vi "FEA_Model_Element_Matrix.vi"(11 "FEA_Model in":refnum<class "FEA_Model.lvclass">) -> (3 "FEA_Model out":refnum<class "FEA_Model.lvclass">)   [LabVIEW 2021, in "FEA_Model.lvclass"]
uses:
  FEA_Model.lvclass
  FEA_Model.lvclass/FEA_Model.ctl
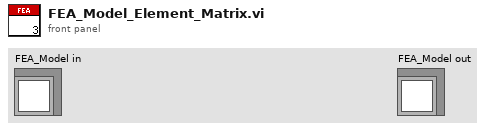
[diagram p1: front panel]
types:
  T1 = cluster{"beam_length":dbl, "youngs_modulus":dbl, "torsion_spring":dbl, "beam_height":dbl, "beam_width":dbl, "beam_density":dbl, "number_of_FEA_nodes":i32, "accelerometer_mass":dbl, "M Matrix":dbl[][], "K Matrix":dbl[][]}
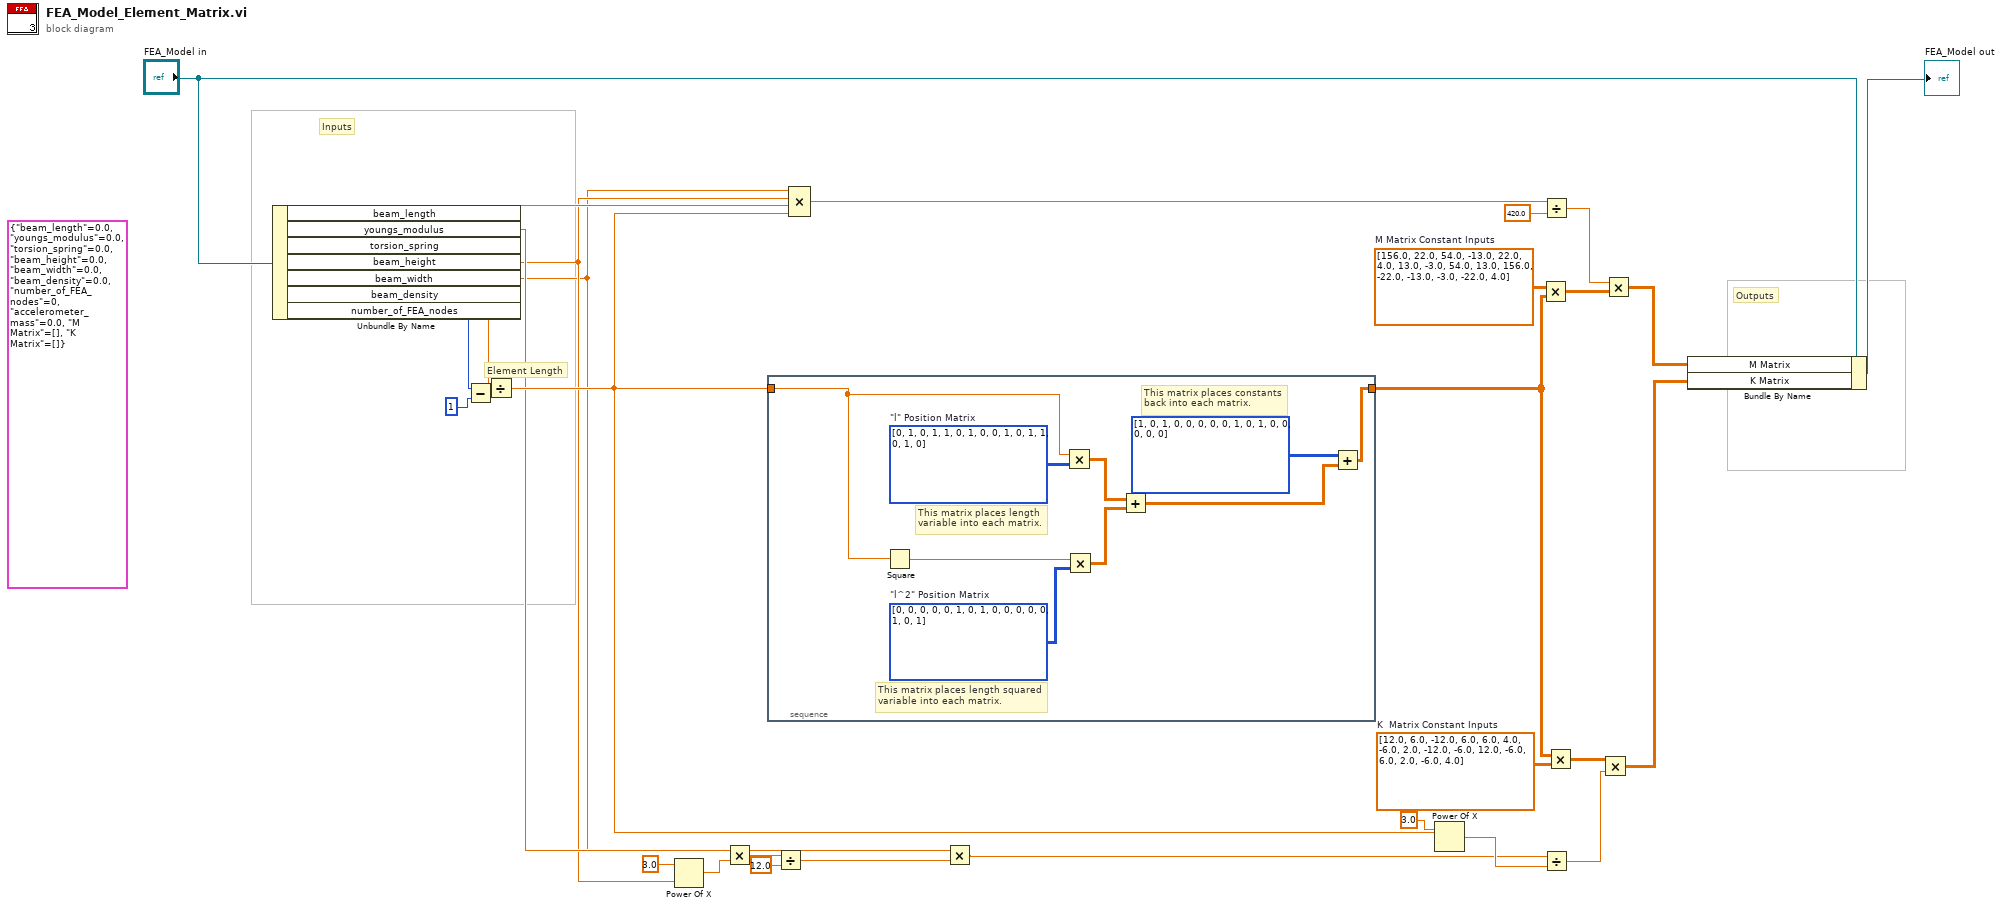
[diagram p0: block diagram]
diagram:
  (unwired) T1 {"beam_length"=0.0, "youngs_modulus"=0.0, "torsion_spring"=0.0, "beam_height"=0.0, "beam_width"=0.0, "beam_density"=0.0, "number_of_FEA_nodes"=0, "accelerometer_mass"=0.0, "M Matrix"=[], "K Matrix"=[]} ("Modeling Parameters")
  w22 = dbl[][] [[12.0, 6.0, -12.0, 6.0], [6.0, 4.0, -6.0, 2.0], [-12.0, -6.0, 12.0, -6.0], [6.0, 2.0, -6.0, 4.0]]  # K  Matrix Constant Inputs
  w27 = dbl[][] [[156.0, 22.0, 54.0, -13.0], [22.0, 4.0, 13.0, -3.0], [54.0, 13.0, 156.0, -22.0], [-13.0, -3.0, -22.0, 4.0]]  # M Matrix Constant Inputs
  # "Outputs"
  # "Element Length"
  # "Inputs"
  n1 = Unbundle By Name("FEA_Model in") -> ("beam_length"=w10:dbl, "youngs_modulus"=w9:dbl, "beam_height"=w6:dbl, "beam_width"=w5:dbl, "beam_density"=w7:dbl, "number_of_FEA_nodes"=w8:i32)  [unwired: 1 out]
  n2 = Subtract(x=w8, y=1) -> (x-y=w26:i32)
  n3 = Divide(x=w10, y=w26) -> (x/y=w15:dbl)
  n4 = Power Of X(1:w6, 2:3.0 ("x")) -> (0:w13:dbl)
  n5 = Multiply(x=w5, y=w13) -> (x*y=w12:dbl)
  n6 = stacked-sequence {
    tunnel: [w37] -> w23
    tunnel: w15 -> [w39]
    frame #0 {
      w32 = i32[][] [[0, 0, 0, 0], [0, 1, 0, 1], [0, 0, 0, 0], [0, 1, 0, 1]]  # "l^2" Position Matrix
      w31 = i32[][] [[0, 1, 0, 1], [1, 0, 1, 0], [0, 1, 0, 1], [1, 0, 1, 0]]  # "l" Position Matrix
      # "This matrix places length squared\nvariable into each matrix."
      # "This matrix places length \nvariable into each matrix."
      # "This matrix places constants\nback into each matrix."
      n7 = Square(x=w39) -> (x^2=w34:dbl)
      n8 = Multiply(x=w39, y=w31) -> (x*y=w33:dbl[][])
      n9 = Multiply(x=w34, y=w32) -> (x*y=w35:dbl[][])
      n10 = Add(x=w33, y=w35) -> (x+y=w38:dbl[][])
      n11 = Add(x=i32[][] [[1, 0, 1, 0], [0, 0, 0, 0], [1, 0, 1, 0], [0, 0, 0, 0]], y=w38) -> (x+y=w37:dbl[][])
    }
  }
  n12 = Divide(x=w12, y=12.0) -> (x/y=w17:dbl)
  n13 = Compound Arithmetic op=MULTIPLY(w5, w6, w7, w15) -> (w28:dbl)
  n14 = Multiply(x=w9, y=w17) -> (x*y=w18:dbl)
  n15 = Power Of X(1:w15, 2:3.0 ("x")) -> (0:w21:dbl)
  n16 = Multiply(x=w27, y=w23) -> (x*y=w29:dbl[][])
  n17 = Divide(x=w28, y=420.0) -> (x/y=w30:dbl)
  n18 = Divide(x=w18, y=w21) -> (x/y=w20:dbl)
  n19 = Multiply(x=w23, y=w22) -> (x*y=w19:dbl[][])
  n20 = Multiply(x=w19, y=w20) -> (x*y=w3:dbl[][])
  n21 = Multiply(x=w30, y=w29) -> (x*y=w4:dbl[][])
  n22 = Bundle By Name(cluster="FEA_Model in", "M Matrix"=w4, "K Matrix"=w3) -> (→"FEA_Model out":refnum<class "FEA_Model.lvclass">)
